vi "example_4.vi"(8 "Error In":errorcluster) -> (0 "Error Out":errorcluster)   [LabVIEW 2014]
panel:
  in  "array in":dbl[](graph)
  out "array out":dbl[](graph)
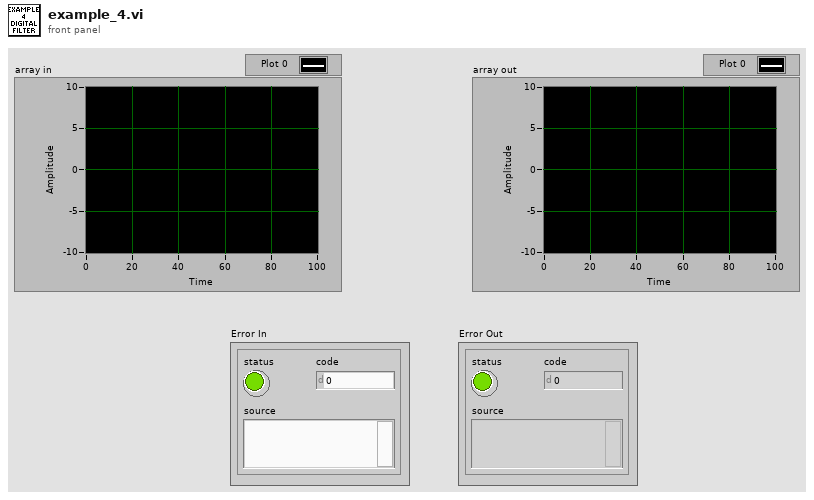
[diagram p1: front panel]
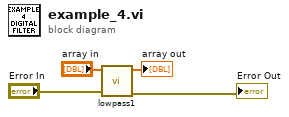
[diagram p0: block diagram]
diagram:
  n1 = call "lowpass1.vi"("Error In"="Error In", "array in"="array in") -> ("Error Out"=→"Error Out":errorcluster, "array out"=→"array out":dbl[])  [unwired: 8 in]
